vi "Galvo Test Harness.vi"() -> ()   [LabVIEW 2014, in "NI Galvo.lvclass"]
uses:
  NI Galvo.lvclass
  Scanning Cluster.ctl
  DAQ/DAQ Parameters.ctl
  DAQ/Trigger Source.ctl
  DAQ/Trigger Slope.ctl
  Type Defs/OCT DAQ Channel Data Type.ctl
  DAQ/Clock Control.ctl
  Galvo.lvclass
  DAQ/DAQ Class.lvclass
panel:
  in  "Boolean":bool
  in  "DAQ Parameters":T1={"Points Per A-Scan"=1024, "A-Scans Per B-Scan"=250, "Number of B-Scans"=1, "A-Scans Per Transfer"=250, "Trigger Voltage"=0.0, "Trigger Source"=enum."External", "Trigger Slope"=enum."Rising", "Channel"=enum."Channel 1", "Clock"=enum."Internal Clock", "Bits per Sample"=0.0, "Range"=0.0}
  in  "Scanning Parameters":T6={"Fast Axis Offset"=0.0, "Slow Axis Offset"=0.0, "Slow Axis Amp"=5.0, "Fast Axis Amp"=5.0, "Scan Pattern"=enum."Raster"} {"Fast Axis Amp" max=20 format="%#.2f"; "Slow Axis Amp" max=20 format="%#.2f"; "Slow Axis Offset" max=10 format="%#.2f"; "Fast Axis Offset" max=10 format="%#.2f"}
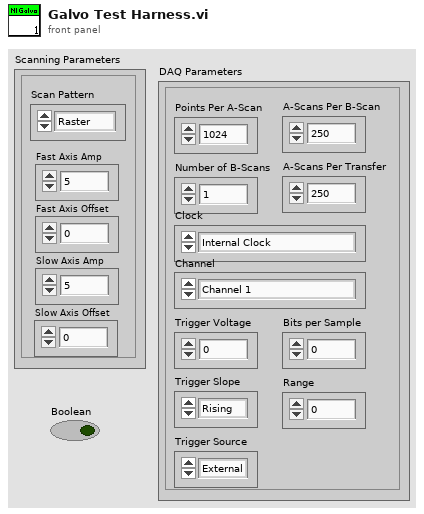
[diagram p1: front panel]
types:
  T1 = typedef "DAQ Class.lvclass/DAQ Parameters.ctl" = cluster{"Points Per A-Scan":u32, "A-Scans Per B-Scan":u32, "Number of B-Scans":u32, "A-Scans Per Transfer":u32, "Trigger Voltage":sgl, "Trigger Source":T2, "Trigger Slope":T3, "Channel":T4, "Clock":T5, "Bits per Sample":dbl, "Range":dbl}
  T2 = typedef "DAQ Class.lvclass/Trigger Source.ctl" = enum16{"External", "Channel A", "Channel B"}
  T3 = typedef "DAQ Class.lvclass/Trigger Slope.ctl" = enum16{"Rising", "Falling"}
  T4 = typedef "OCT DAQ Channel Data Type.ctl" = enum16{"Channel 1", "Channel 2", "Channel 1 and 2"}
  T5 = typedef "DAQ Class.lvclass/Clock Control.ctl" = enum16{"Internal Clock", "External Clock"}
  T6 = typedef "Galvo.lvclass/Scanning Cluster.ctl" = cluster{"Fast Axis Offset":sgl, "Slow Axis Offset":sgl, "Slow Axis Amp":sgl, "Fast Axis Amp":sgl, "Scan Pattern":enum16{"Raster"}}
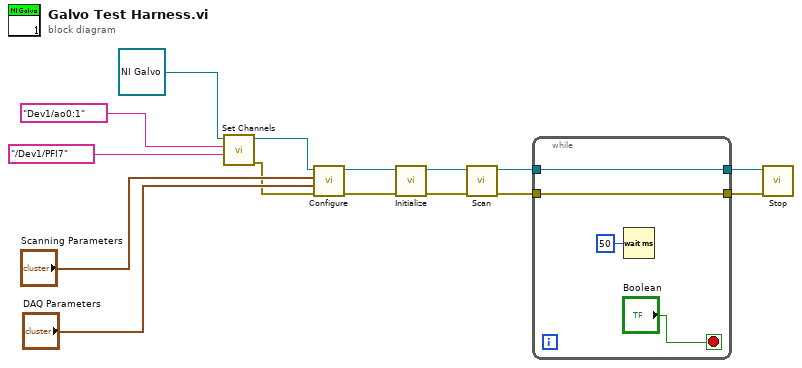
[diagram p0: block diagram]
diagram:
  n1 = call-dynamic "Set Channels.vi"("Trigger Source"=tag "/Dev1/PFI7", "Analog Output"=tag "Dev1/ao0:1", "NI Galvo in"=refnum<class "NI Galvo.lvclass"> refnum ("NI Galvo.lvclass")) -> ("error out"=w11:errorcluster, "NI Galvo out"=w10:refnum<class "NI Galvo.lvclass">)  [unwired: 7 in]
  n2 = call-dynamic "Configure.vi"("error in (no error)"=w11, "DAQ Parameters"="DAQ Parameters", "Scanning Parameters"="Scanning Parameters", "NI Galvo in"=w10) -> ("error out"=w13:errorcluster, "NI Galvo out"=w12:refnum<class "NI Galvo.lvclass">)  [unwired: 6 in]
  n3 = call-dynamic "Initialize.vi"("error in (no error)"=w13, "NI Galvo in"=w12) -> ("error out"=w5:errorcluster, "NI Galvo out"=w6:refnum<class "NI Galvo.lvclass">)  [unwired: 8 in]
  n4 = call-dynamic "Scan.vi"("error in (no error)"=w5, "NI Galvo in"=w6) -> ("error out"=w4:errorcluster, "NI Galvo out"=w3:refnum<class "NI Galvo.lvclass">)  [unwired: 8 in]
  n5 = while {
    tunnel: w4 -> [w18]
    tunnel: w3 -> [w19]
    tunnel: [w19] -> w2
    tunnel: [w18] -> w1
    stop <- "Boolean" stop-if-true
    n6 = Wait (ms)(milliseconds to wait=u32 50) -> ()  [unwired: 1 out]
  }
  n7 = call-dynamic "Stop.vi"("error in (no error)"=w1, "NI Galvo in"=w2) -> ()  [unwired: 8 in, 2 out]
